vi "mediaBalls_v2.vi"(7 "cameras array":dbl[](array[numeric]), 9 "Field Size":T2, 10 "grSim?":bool=TRUE, 11 "Array Ball Pose + CamID":T1(array[cluster])) -> (2 "No cameras?":bool, 3 "Ball out":cluster{"x":dbl, "y":dbl})   [LabVIEW 2023]
panel:
  out "Array":i32[](array[numeric])
  in  "Cam Intersection Widht":u32=6
  in  "Cam Intersection Lenght":u32=6
  in  "cluster":cluster{"x":dbl, "y":dbl}
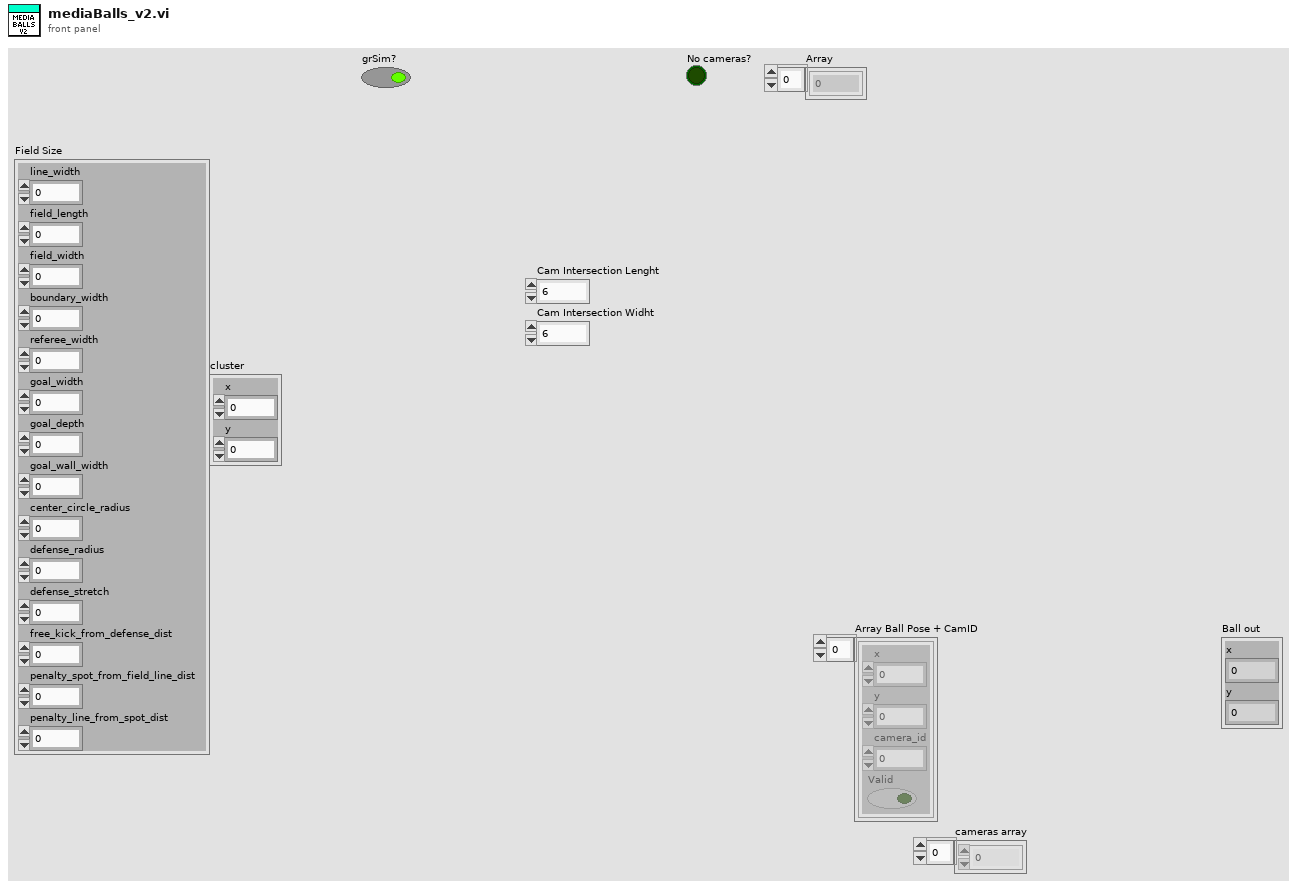
[diagram p1: front panel]
types:
  T1 = cluster{"x":sgl, "y":sgl, "camera_id":u32, "Valid":bool}[]
  T2 = cluster{"line_width":u32, "field_length":u32, "field_width":u32, "boundary_width":u32, "referee_width":u32, "goal_width":u32, "goal_depth":u32, "goal_wall_width":u32, "center_circle_radius":u32, "defense_radius":u32, "defense_stretch":u32, "free_kick_from_defense_dist":u32, "penalty_spot_from_field_line_dist":u32, "penalty_line_from_spot_dist":u32}
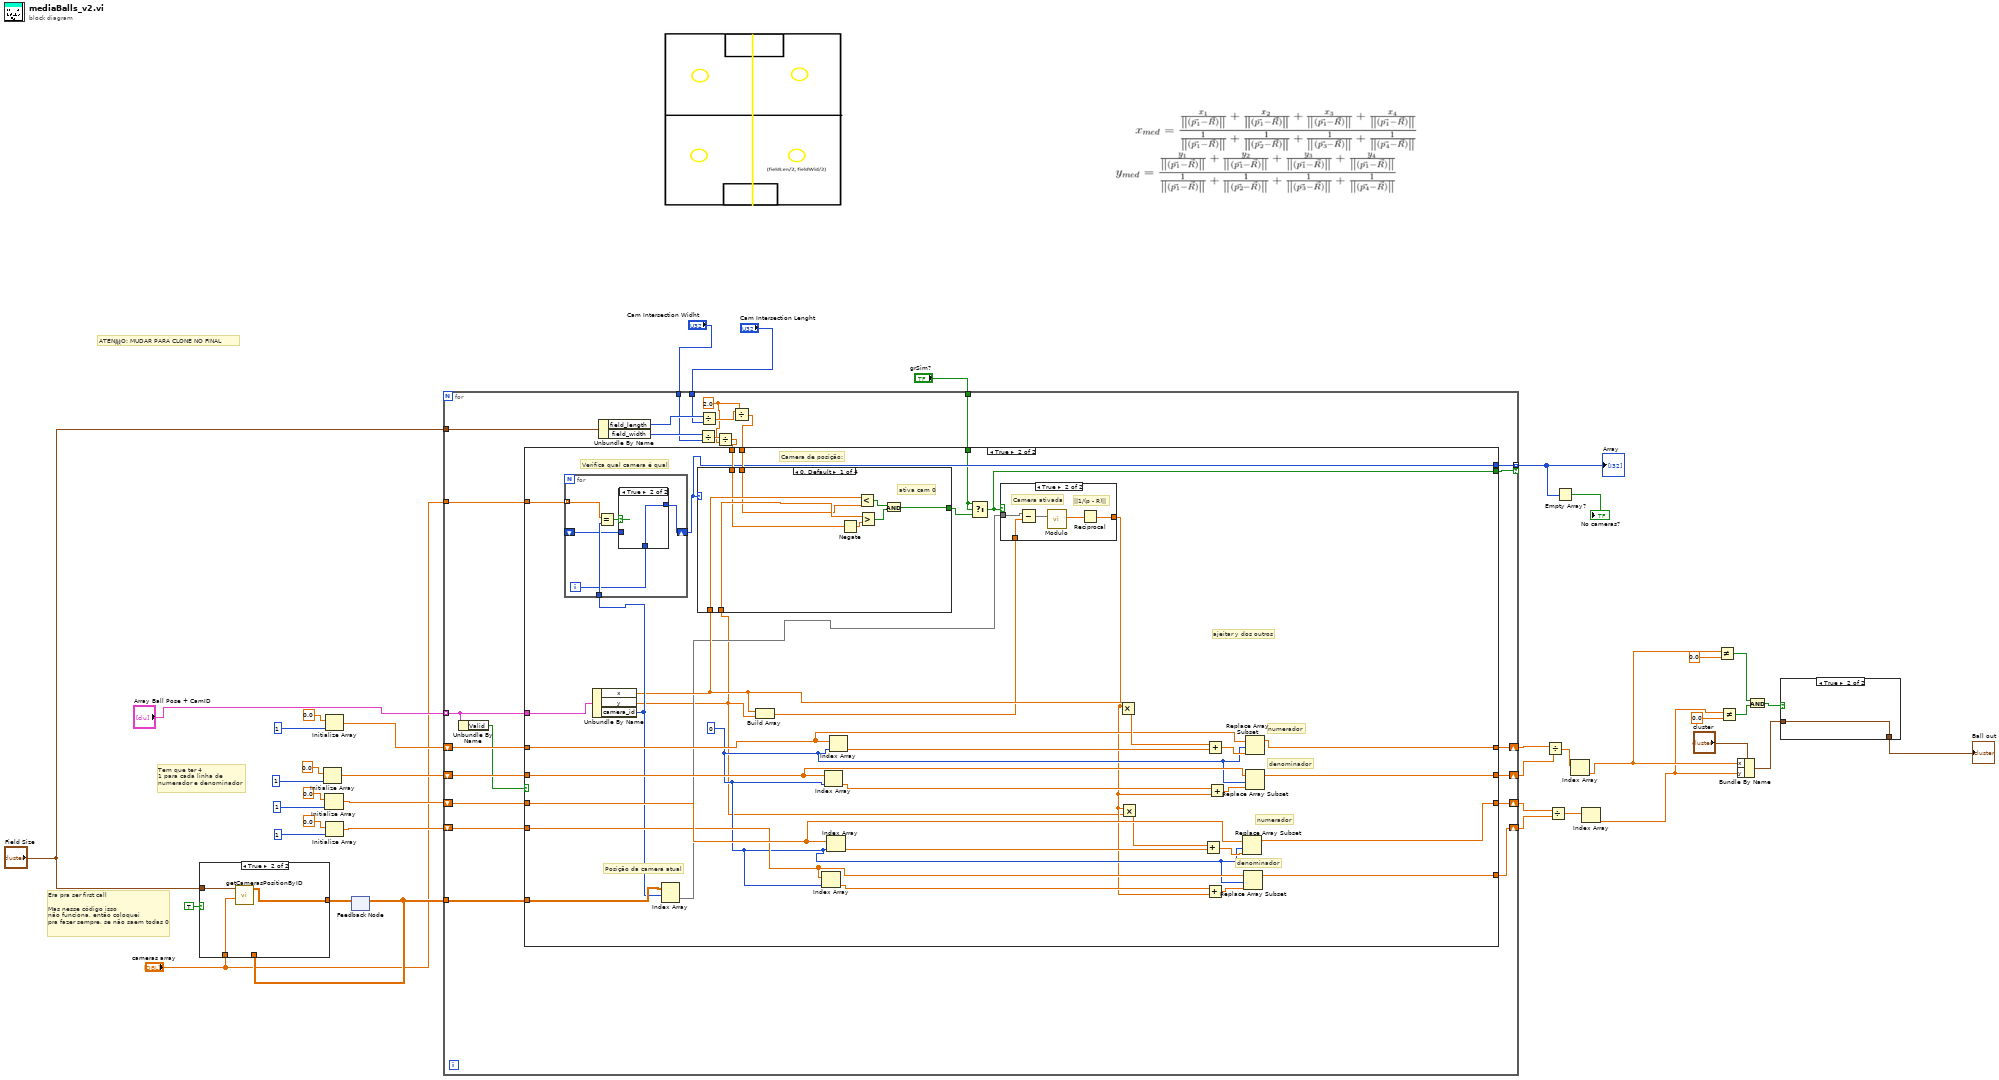
[diagram p0: block diagram]
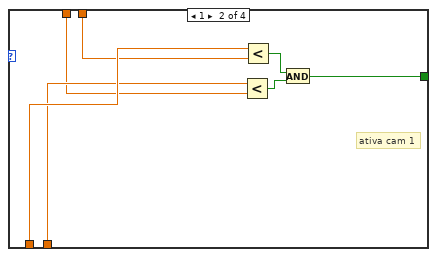
[diagram p5: hidden frame]
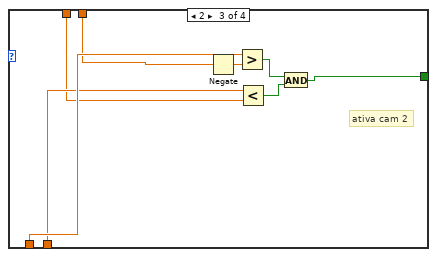
[diagram p6: hidden frame]
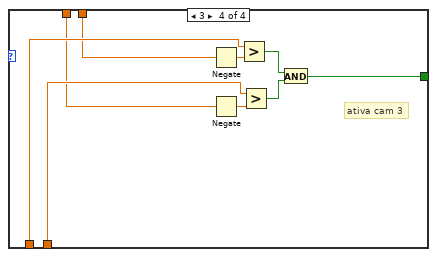
[diagram p7: hidden frame]
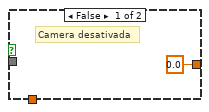
[diagram p9: hidden frame]
diagram:
  # "Era pra ser first call\n\nMas nesse código isso\nnão funciona, então coloquei\npra fazer sempre, se não saem todas 0"
  # "Tem que ter 4\n1 para cada linha de\nnumerador e denominador"
  # "ATEN敲O: MUDAR PARA CLONE NO FINAL"
  n1 = Initialize Array(0.0 ("element"), 1 ("dimension size")) -> (w30:dbl[])
  n2 = Initialize Array(0.0 ("element"), 1 ("dimension size")) -> (w29:dbl[])
  n3 = Initialize Array(0.0 ("element"), 1 ("dimension size")) -> (w31:dbl[])
  n4 = Initialize Array(0.0 ("element"), 1 ("dimension size")) -> (w28:dbl[])
  n5 = feedback #1() -> (w9:dbl[][])  [unwired: 1 in]
  n6 = case shown="True" TRUE {
    tunnel: "Field Size" -> [_ w43]
    tunnel: [w40 w42] -> w10
    tunnel: w9 -> [w40 _]
    tunnel: "cameras array" -> [_ w41]
    frame False {
    }
    frame True {
      n7 = call "getCamerasPositionByID.vi"("cameras id"=w41, "Field Size 2"=w43) -> ("Cameras Positions"=w42:dbl[][])  [unwired: 9 in]
    }
  }
  n8 = feedback-in #1(w10) -> ()
  n9 = for {
    tunnel: "Array Ball Pose + CamID" -> [w45] mode=indexing
    tunnel: w9 -> [w68]
    shift-right: [w67] -> w27
    shift-left: w31 -> [w61]
    shift-right: [w66] -> w26
    shift-left: w30 -> [w60]
    shift-right: [w65] -> w25
    shift-left: w29 -> [w63]
    shift-right: [w64] -> w24
    shift-left: w28 -> [w62]
    tunnel: "cameras array" -> [w59]
    tunnel: "Cam Intersection Widht" -> [w56]
    tunnel: "Cam Intersection Lenght" -> [w55]
    tunnel: "Field Size" -> [w54]
    tunnel: "grSim?" -> [w53]
    tunnel: [w52] -> w5 mode=indexing if=w51
    w46 = 2.0
    n10 = Unbundle By Name(w45) -> ("Valid"=w44:bool)
    n11 = Unbundle By Name(w54) -> ("field_length"=w58:u32, "field_width"=w57:u32)
    n12 = Divide(x=w57, y=w56) -> (x/y=w48:dbl)
    n13 = Divide(x=w58, y=w55) -> (x/y=w50:dbl)
    n14 = Divide(x=w48, y=w46) -> (x/y=w47:dbl)
    n15 = Divide(x=w50, y=w46) -> (x/y=w49:dbl)
    n16 = case shown="True" w44 {
      tunnel: w68 -> [_ w106]
      tunnel: [w72 w96] -> w67
      tunnel: [w71 w95] -> w66
      tunnel: [w70 w94] -> w65
      tunnel: [w69 w93] -> w64
      tunnel: w63 -> [w70 w92]
      tunnel: w62 -> [w69 w91]
      tunnel: w61 -> [w72 w90]
      tunnel: w60 -> [w71 w89]
      tunnel: w45 -> [_ w86]
      tunnel: w59 -> [_ w84]
      tunnel: w47 -> [_ w83]
      tunnel: w49 -> [_ w82]
      tunnel: w53 -> [_ w75]
      tunnel: [_ w76] -> w52
      tunnel: [_ w73] -> w51
      frame False {
      }
      frame True {
        w88 = 0 ("index")
        # "Verifica qual camera é qual"
        # "Camera de posição:"
        # "ajeitar y dos outros"
        # "denominador"
        # "numerador"
        # "denominador"
        # "numerador"
        # "Posição da camera atual"
        n17 = Unbundle By Name(w86) -> ("x"=w81:sgl, "y"=w77:sgl, "camera_id"=w85:u32)
        n18 = for {
          tunnel: w85 -> [w144]
          shift-right: [w141] -> w76
          shift-left: _ -> [w140]
          tunnel: w84 -> [w139] mode=indexing
          i -> [w142]
          n19 = Equal?(x=w139, y=w144) -> (x = y?=w143:bool)
          n20 = case shown="True" w143 {
            tunnel: w142 -> [_ w146]
            tunnel: [w145 w146] -> w141
            tunnel: w140 -> [w145 _]
            frame False {
            }
            frame True {
            }
          }
        }
        n21 = Index Array(array=w106, index (row)=w85) -> (element=w80:dbl[])  [unwired: 1 in]
        n22 = case shown="0, Default" w76 {
          tunnel: w81 -> [w111 w119 w126 w134]
          tunnel: w77 -> [w110 w118 w125 w133]
          tunnel: [w107 w115 w122 w130] -> w74
          tunnel: w82 -> [w109 w117 w124 w132]
          tunnel: w83 -> [w108 w116 w123 w131]
          frame 0, Default {
            # "ativa cam 0"
            n23 = Negate(x=w108) -> (-x=w112:dbl)
            n24 = Less?(x=w111, y=w109) -> (x < y?=w114:bool)
            n25 = Greater?(x=w110, y=w112) -> (0:w113:bool)
            n26 = And(x=w114, y=w113) -> (x .and. y?=w107:bool)
          }
          frame 1 {
            # "ativa cam 1"
            n27 = Less?(x=w118, y=w116) -> (x < y?=w121:bool)
            n28 = Less?(x=w119, y=w117) -> (x < y?=w120:bool)
            n29 = And(x=w120, y=w121) -> (x .and. y?=w115:bool)
          }
          frame 2 {
            # "ativa cam 2"
            n30 = Negate(x=w124) -> (-x=w129:dbl)
            n31 = Greater?(x=w126, y=w129) -> (0:w128:bool)
            n32 = Less?(x=w125, y=w123) -> (x < y?=w127:bool)
            n33 = And(x=w128, y=w127) -> (x .and. y?=w122:bool)
          }
          frame 3 {
            # "ativa cam 3"
            n34 = Negate(x=w132) -> (-x=w138:dbl)
            n35 = Negate(x=w131) -> (-x=w137:dbl)
            n36 = Greater?(x=w134, y=w138) -> (0:w135:bool)
            n37 = Greater?(x=w133, y=w137) -> (0:w136:bool)
            n38 = And(x=w135, y=w136) -> (x .and. y?=w130:bool)
          }
        }
        n39 = Build Array(w81, w77) -> (w79:sgl[])
        n40 = Index Array(array=w91, index=w88) -> (element=w97:dbl)
        n41 = Index Array(array=w89, index=w88) -> (element=w99:dbl)
        n42 = Index Array(array=w92, index=w88) -> (element=w98:dbl)
        n43 = Index Array(array=w90, index=w88) -> (element=w100:dbl)
        n44 = Select(t=w75, s=w75, f=w74) -> (s? t:f=w73:bool)
        n45 = case shown="True" w73 {
          tunnel: [0.0 w151] -> w78
          tunnel: w80 -> [_ w150]
          tunnel: w79 -> [_ w149]
          frame False {
            # "Camera desativada"
          }
          frame True {
            # "Camera ativada"
            # "||1/(p - R)||"
            n46 = Subtract(x=w150, y=w149) -> (x-y=w148:dbl[])
            n47 = call "Modulo.vi"("2D vector"=w148) -> ("Modulo"=w152:dbl)  [unwired: 10 in]
            n48 = Reciprocal(x=w152) -> (1/x=w151:dbl)
          }
        }
        n49 = Multiply(x=w78, y=w81) -> (x*y=w105:dbl)
        n50 = Multiply(x=w78, y=w77) -> (x*y=w87:dbl)
        n51 = Add(x=w87, y=w98) -> (x+y=w102:dbl)
        n52 = Add(x=w97, y=w78) -> (x+y=w101:dbl)
        n53 = Add(x=w105, y=w100) -> (x+y=w104:dbl)
        n54 = Add(x=w99, y=w78) -> (x+y=w103:dbl)
        n55 = Replace Array Subset(array=w92, new element=w102, index=w88) -> (w94:dbl[])
        n56 = Replace Array Subset(array=w91, new element=w101, index=w88) -> (w93:dbl[])
        n57 = Replace Array Subset(array=w90, new element=w104, index=w88) -> (w96:dbl[])
        n58 = Replace Array Subset(array=w89, new element=w103, index=w88) -> (w95:dbl[])
      }
    }
  }
  "Array" <- w5
  n59 = Divide(x=w27, y=w26) -> (x/y=w16:dbl[])
  n60 = Divide(x=w25, y=w24) -> (x/y=w14:dbl[])
  n61 = Empty Array?(array=w5) -> (empty?=→"No cameras?":bool)
  n62 = Index Array(array=w16) -> (element=w15:dbl)  [unwired: 1 in]
  n63 = Index Array(array=w14) -> (element=w13:dbl)  [unwired: 1 in]
  n64 = Not Equal?(x=w15, y=0.0) -> (x != y?=w21:bool)
  n65 = Not Equal?(x=w13, y=0.0) -> (x != y?=w20:bool)
  n66 = Bundle By Name(cluster="cluster", "x"=w15, "y"=w13) -> (w18:cluster{"x":dbl, "y":dbl})
  n67 = And(x=w21, y=w20) -> (x .and. y?=w19:bool)
  n68 = case shown="True" w19 {
    tunnel: [w153 w154] -> w12
    tunnel: w18 -> [w153 w154]
    frame False {
    }
    frame True {
    }
  }
  "Ball out" <- w12
